vi "Strings and Values.vi"(8 "error in (no error)":errorcluster, 11 "Predefined Values in":refnum<class "Predefined Values.lvclass">) -> (0 "error out":errorcluster, 2 "Strings And Values []":T1, 3 "Predefined Values out":refnum<class "Predefined Values.lvclass">)   [LabVIEW 2020, in "Dynamic Combobox.lvlib" / "Predefined Values.lvclass"]
uses:
  Predefined Values.lvclass
  <vilib>/Utility/miscctls.llb/LVComboBoxStrsAndValuesArrayTypeDef.ctl
  Predefined Values.lvclass/Predefined Values.ctl
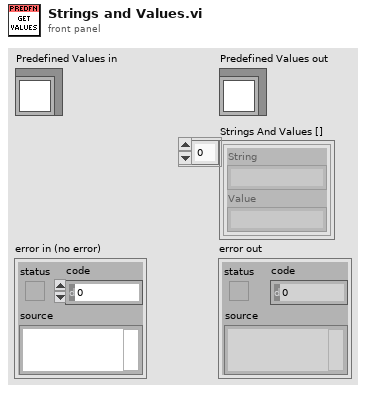
[diagram p1: front panel]
types:
  T1 = typedef "LVComboBoxStrsAndValuesArrayTypeDef.ctl" = cluster{"String":string, "Value":string}[]
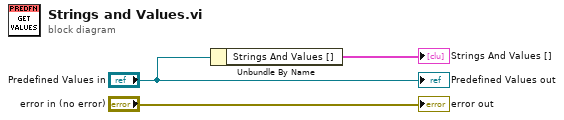
[diagram p0: block diagram]
diagram:
  n1 = Unbundle By Name("Predefined Values in") -> ("Strings And Values []"=→"Strings And Values []":T1)
  "error out" <- "error in (no error)"
  "Predefined Values out" <- "Predefined Values in"
